vi "init.vi"(8 "error in (no error)":errorcluster, 11 "Mensaje Actor in":refnum<class "Mensaje Actor.lvclass">) -> (0 "error out":errorcluster, 3 "Mensaje Actor out":refnum<class "Mensaje Actor.lvclass">)   [LabVIEW 2019, in "Mensaje Actor.lvlib"]
uses:
  Mensaje Actor.lvlib
  Mensaje Actor.lvclass
  C:/Program Files (x86)/National Instruments/LabVIEW 2019/vi.lib/ActorFramework/Actor/Actor.lvclass
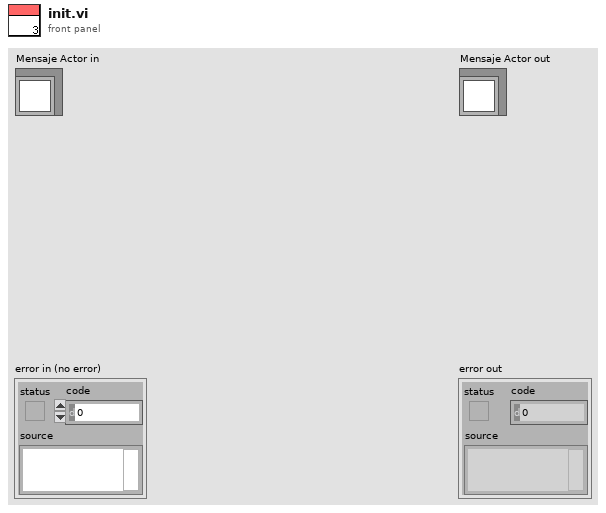
[diagram p1: front panel]
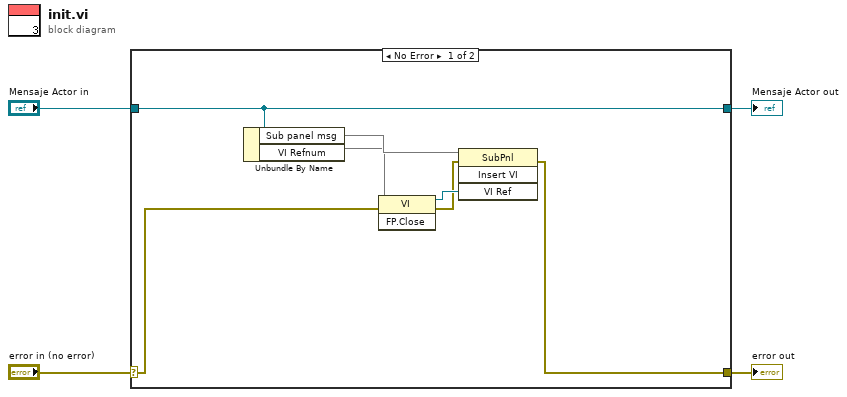
[diagram p0: block diagram]
diagram:
  n1 = case shown="No Error" "error in (no error)" {
    selector: "error in (no error)" -> [w6 w13]
    tunnel: [w5 w13] -> w3
    tunnel: [w11 w12] -> w1
    tunnel: "Mensaje Actor in" -> [w11 w12]
    frame No Error {
      n2 = Unbundle By Name(w11) -> ("Sub panel msg"=w8, "VI Refnum"=w7)
      n3 = invoke class="VI" method="FP.Close"(reference=w7, error in=w6) -> (reference out=w10:refnum<vi>, error out=w9:errorcluster)  [unwired: 1 in, 1 out]
      n4 = invoke class="SubPnl" method="Insert VI"(reference=w8, error in=w9, "VI Ref"=w10) -> (error out=w5:errorcluster)  [unwired: 1 in, 3 out]
    }
    frame Error {
    }
  }
  "error out" <- w3
  "Mensaje Actor out" <- w1
